vi "Average.vi"(8 "error in (no error)":errorcluster, 10 "Configure":T1={"X Low"=0.05, "X High"=0.5, "X Step"=0.01, "Fake Point"=0.05} {"Fake Point" format="%#_6p"; "X Step" format="%#_6p"; "X High" format="%#_6p"; "X Low" format="%#_6p"}, 11 "XY-data":cluster{"X-array":dbl[], "Y-array":dbl[]}[](array[cluster]) {"Y-array" format="%.2p"; "X-array" format="%.2p"}) -> (0 "error out":errorcluster, 2 "Averaged XY-data out":cluster{"X-array":dbl[], "Y-array":dbl[]} {"Y-array" format="%.2p"; "X-array" format="%.2p"}, 3 "XY-data out":cluster{"X-array":dbl[], "Y-array":dbl[]}[](array[cluster]) {"Y-array" format="%.2p"; "X-array" format="%.2p"})   [LabVIEW 2016, in "xy_utilities.lvlib"]
doc: "Calculates the <b>Mean</b> of the y arrays in <b>XY-data</b> at x values defined by the <b>Configure</b> Cluster.\n\n<b>XY-data</b> is not assumed to have commensurate x values or sampling; therefore interpolation is performed before averaging.\n\nThe <b>Configure</b> cluster is used to define:\n<b>X Low</b>: Starting x value for interpolation. May lie outside of the input x array range.\n<b>X High</b>: Ending x value for interpolation. May lie outside of the input x array range.\n<b>X Step</b>: Interpolation value.\n<b>Fake Point</b>: Value added to the y array for x values outside of the x array input range.\n\nNote that this VI returns two types of data:\n<b>XY-data out</b> is the original input data array <b>XY-data</b>.\n<b>Averaged XY-data out</b> is a single containing the averaged XY-data.\n\nNote also that this is NOT a polymorphic VI. It will only work for an input that is an array of XY-data."
uses:
  xy_utilities.lvlib
  <vilib>/Analysis/baseanly.llb/Mean (DBL).vi
  <vilib>/Analysis/NI_AALBase.lvlib
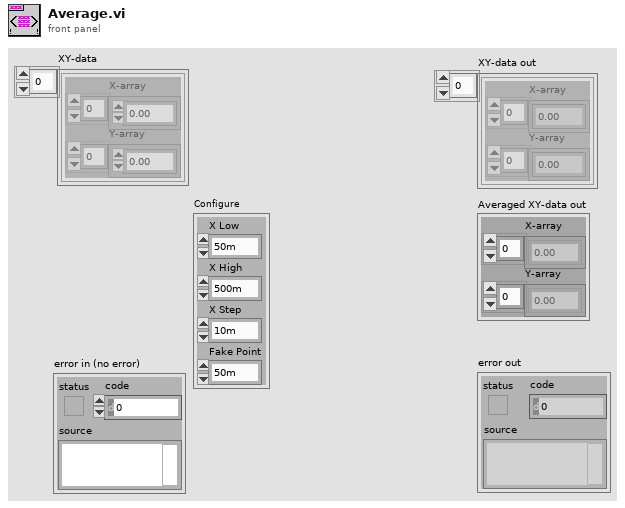
[diagram p1: front panel]
types:
  T1 = cluster{"X Low":dbl, "X High":dbl, "X Step":dbl, "Fake Point":dbl}
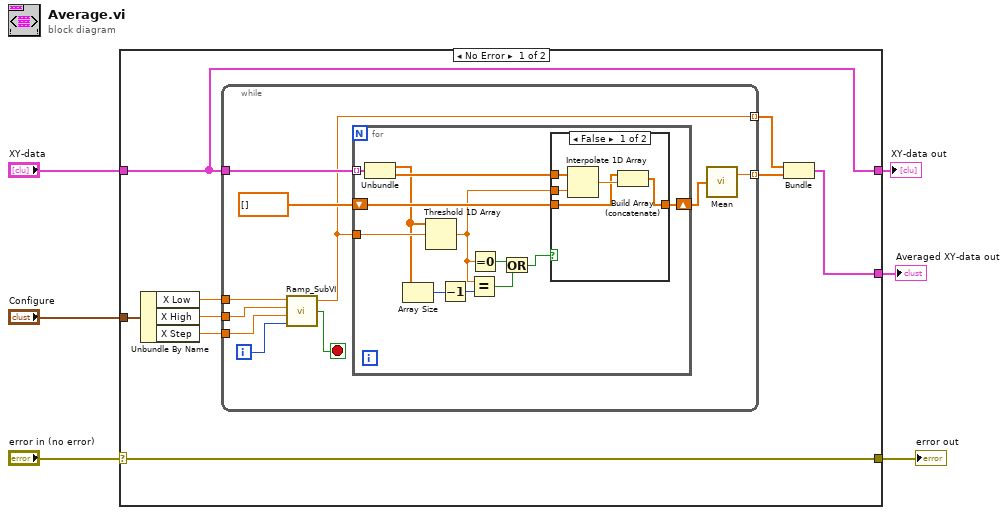
[diagram p0: block diagram]
diagram:
  n1 = case shown="No Error" "error in (no error)" {
    selector: "error in (no error)" -> [w14 w44]
    tunnel: [w7 w45] -> w6
    tunnel: "XY-data" -> [w7 w45]
    tunnel: [w14 w44] -> w4
    tunnel: "Configure" -> [w13 _]
    tunnel: [w8 _] -> w1
    frame No Error {
      n2 = Unbundle By Name(w13) -> ("X Low"=w12:dbl, "X High"=w11:dbl, "X Step"=w9:dbl)
      n3 = while {
        tunnel: [w24] -> w15 mode=indexing
        tunnel: [w21] -> w10 mode=indexing
        tunnel: w7 -> [w22]
        tunnel: w12 -> [w20]
        tunnel: w11 -> [w19]
        tunnel: w9 -> [w18]
        i -> [w17]
        stop <- w16 stop-if-true
        n4 = call <userlib>:"Ramp_SubVI.vi"("index"=w17, "step"=w18, "end"=w19, "start"=w20) -> ("Stop?"=w16:bool, "Numeric"=w21:dbl)  [unwired: 1 in]
        n5 = for {
          tunnel: w22 -> [w37] mode=indexing
          shift-right: [w36] -> w23
          shift-left: dbl[] [] -> [w35]
          tunnel: w21 -> [w34]
          n6 = Unbundle(w37) -> ("X-array"=w27:dbl[], "Y-array"=w28:dbl[])
          n7 = Array Size(array=w27) -> (size(s)=w30:i32)
          n8 = Threshold 1D Array(2:w34, 3:w27) -> (0:w32:dbl)  [unwired: 1 in]
          n9 = Decrement(x=w30) -> (x-1=w29:i32)
          n10 = Equal?(x=w32, y=w29) -> (x = y?=w31:bool)
          n11 = Equal To 0?(x=w32) -> (x = 0?=w33:bool)
          n12 = Or(x=w33, y=w31) -> (x .or. y?=w26:bool)
          n13 = case shown="False" w26 {
            tunnel: [w40 w43] -> w36
            tunnel: w32 -> [w42 _]
            tunnel: w28 -> [w41 _]
            tunnel: w35 -> [w38 w43]
            frame False {
              n14 = Interpolate 1D Array(1:w42, 2:w41) -> (0:w39:dbl)
              n15 = Build Array (concatenate)(w38, w39) -> (w40:dbl[])
            }
            frame True {
            }
          }
        }
        n16 = call-poly <vilib>:"Mean.vi"("X"=w23) -> ("mean"=w24:dbl)  [unwired: 1 out]
      }
      n17 = Bundle(w10, w15) -> (w8:cluster{dbl[], dbl[]})  [unwired: 1 in]
    }
    frame Error {
    }
  }
  "XY-data out" <- w6
  "error out" <- w4
  "Averaged XY-data out" <- w1
